vi "SymMatrix EigenVectors and Values.vi"(0 "Input Matrix":T2, 1 "output option":T1=1 items=["Eigenvalues", "Eigenvalues & Vectors"]) -> (2 "Eigenvalue":dbl[](array[numeric]), 3 "Eigenvector":T2, 4 "error":i32)   [LabVIEW 2020, in "NI_AALBase.lvlib"]
uses:
  <vilib>/Analysis/NI_AALBase.lvlib
  <vilib>/Analysis/Matrix/Datatypes/RealMatrix.ctl
  <vilib>/Analysis/7linalg.llb/Eigenvalue and Vectors Output Option.ctl
  <resource>/lvanlys.dll
  <vilib>/Analysis/Matrix/NI_Matrix.lvlib
  <vilib>/Analysis/NI_AALPro.lvlib
panel:
  # "SymMatrix EigenVectors and Values"
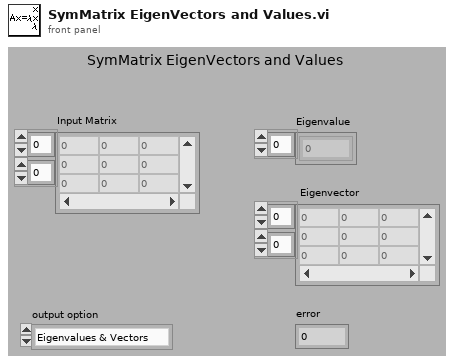
[diagram p1: front panel]
types:
  T1 = typedef "NI_AALPro.lvlib/Eigenvalue and Vectors Output Option.ctl" = i32
  T2 = typedef "NI_Matrix.lvlib/RealMatrix.ctl" = dbl[][]
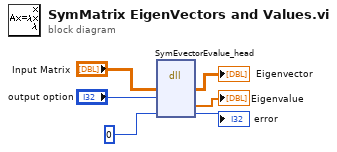
[diagram p0: block diagram]
diagram:
  n1 = dll-call lib="e:/builds/penguin/labview/branches/2020/dev/dist/resource/lvanlys.*" fn="SymEvectorEvalue_head"("Input Matrix"="Input Matrix", "output option"="output option", 0) -> ("Input Matrix"=→"Eigenvector":T2, "Eigenvalue"=→"Eigenvalue":dbl[], →"error":i32)  [unwired: 6 in, 2 out]
